vi "Get Group List.vi"(8 "error in":errorcluster, 11 "TDMS in":refnum<class "TDMS.lvclass">) -> (0 "error out":errorcluster, 2 "group names":string[](array[string]), 3 "TDMS out":refnum<class "TDMS.lvclass">)   [LabVIEW 2019, in "TDMS.lvlib" / "TDMS.lvclass"]
uses:
  TDMS.lvclass
  TDMS.lvclass/TDMS.ctl
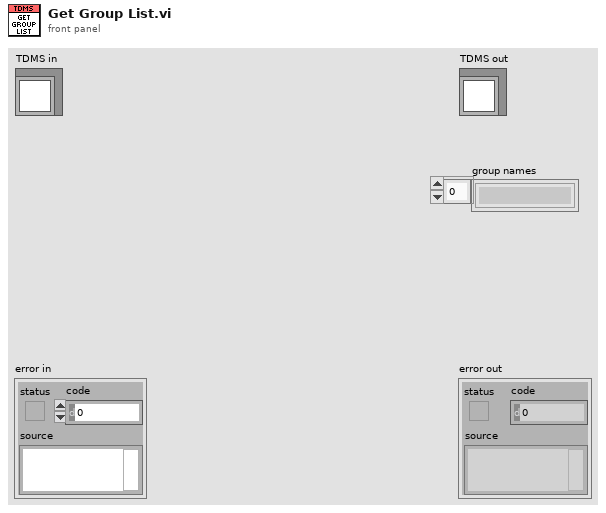
[diagram p1: front panel]
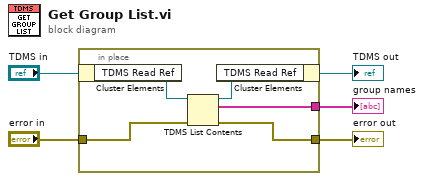
[diagram p0: block diagram]
diagram:
  n1 = in-place {
    in-place-border: "error in" -> [w8]
    in-place-border: [w7] -> w2
    in-place-border: [w6] -> w1
    n2 = in-place-cluster #1("TDMS in") -> ("TDMS Read Ref"=w10:refnum<k34>)
    n3 = TDMS List Contents(4:w8, 7:w10) -> (0:w7:errorcluster, 2:w6:string[], 3:w9:refnum<k34>)  [unwired: 1 in, 1 out]
    n4 = in-place-cluster #1("TDMS Read Ref"=w9) -> (→"TDMS out":refnum<class "TDMS.lvclass">)
  }
  "error out" <- w2
  "group names" <- w1
